vi "event callback.vi"(8 "error in":errorcluster, 10 "User paramter":refnum<queue>, 11 "event data":refnum<k24>) -> (0 "error out":errorcluster, 3 "queue out":refnum<queue>)   [LabVIEW 2020, in "FileCopyEventBased.lvclass"]
uses:
  FileCopyEventBased.lvclass
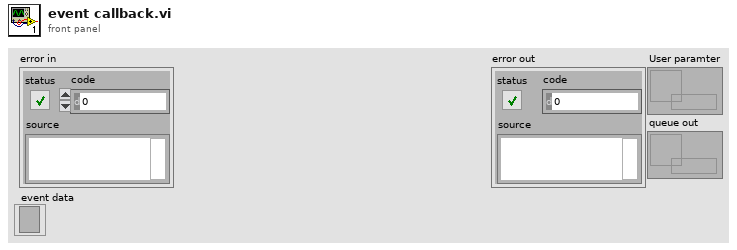
[diagram p1: front panel]
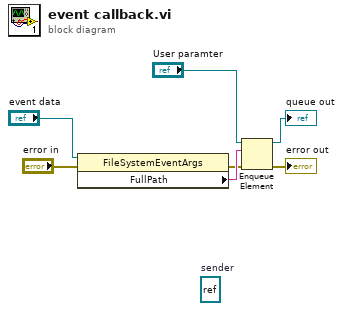
[diagram p0: block diagram]
diagram:
  (unwired) refnum<k24> refnum  # sender
  n1 = property class="FileSystemEventArgs"(reference="event data", error in="error in") -> (error out=w2:errorcluster, "FullPath"=w5:string)  [unwired: 1 out]
  n2 = Enqueue Element(queue="User paramter", element=w5, error in (no error)=w2) -> (queue out=→"queue out":refnum<queue>, error out=→"error out":errorcluster)  [unwired: 1 in, 1 out]
